vi "Parse Error XML.vi"(9 "Code Tag Value":string, 10 "Error XML":string, 11 "AWS Core":refnum<class "IoT Session.lvclass">) -> (1 "Error Description Override":string, 2 "Error Code":i32, 3 "Warning":bool)   [LabVIEW 2015, in "NI_AWS_IoT.lvlib" / "IoT Session.lvclass"]
uses:
  IoT Session.lvclass
  Core/HTTP Request/HTTP Request.lvclass
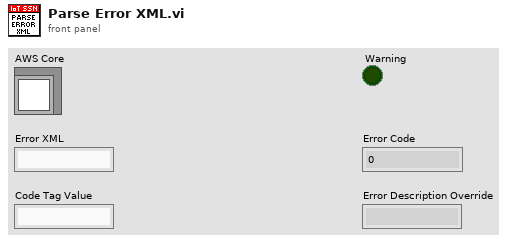
[diagram p1: front panel]
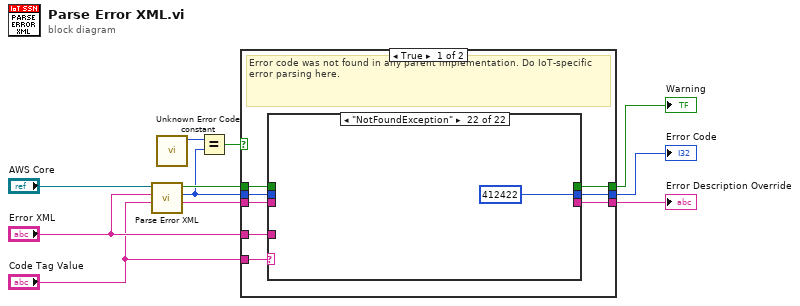
[diagram p0: block diagram]
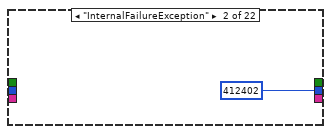
[diagram p3: hidden frame]
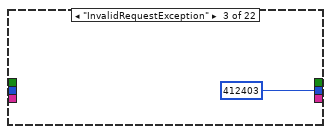
[diagram p4: hidden frame]
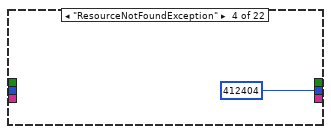
[diagram p5: hidden frame]
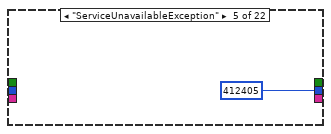
[diagram p6: hidden frame]
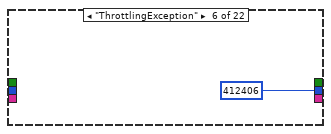
[diagram p7: hidden frame]
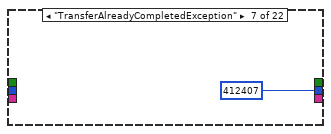
[diagram p8: hidden frame]
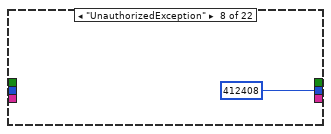
[diagram p9: hidden frame]
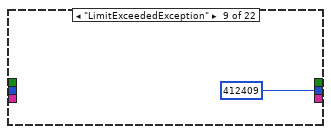
[diagram p10: hidden frame]
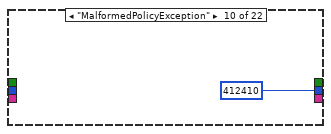
[diagram p11: hidden frame]
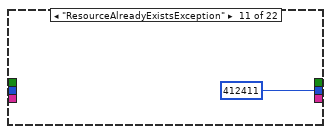
[diagram p12: hidden frame]
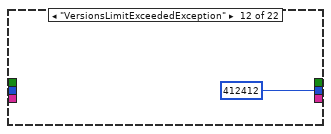
[diagram p13: hidden frame]
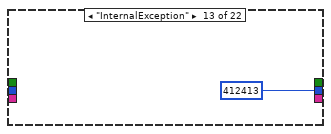
[diagram p14: hidden frame]
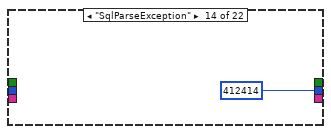
[diagram p15: hidden frame]
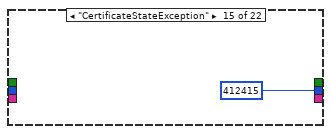
[diagram p16: hidden frame]
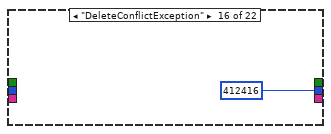
[diagram p17: hidden frame]
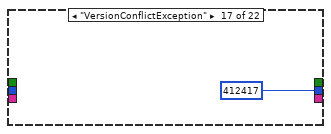
[diagram p18: hidden frame]
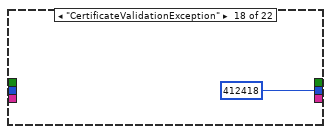
[diagram p19: hidden frame]
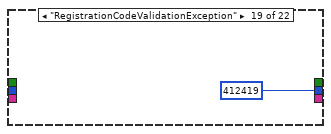
[diagram p20: hidden frame]
diagram:
  n1 = call-parent "Parse Error XML.vi"("Code Tag Value"="Code Tag Value", "Error XML"="Error XML", "AWS Core"="AWS Core") -> ("Error Description Override"=w6:string, "Error Code"=w7:i32, "Warning"=w8:bool)  [unwired: 6 in]
  n2 = call "Unknown Error Code constant.vi"() -> ("AWS Unknown Error Code value"=w10:i32)  [unwired: 11 in]
  n3 = Equal?(x=w10, y=w7) -> (x = y?=w9:bool)
  n4 = case shown="True" w9 {
    tunnel: w8 -> [w17 w46]
    tunnel: w6 -> [w15 w45]
    tunnel: [w14 w46] -> w1
    tunnel: [w12 w45] -> w3
    tunnel: [w13 w44] -> w2
    tunnel: "Error XML" -> [w18 _]
    tunnel: "Code Tag Value" -> [w19 _]
    tunnel: w7 -> [w16 w44]
    frame True {
      # "Error code was not found in any parent implementation. Do IoT-specific error parsing here."
      n5 = case shown="\"NotFoundException\"" w19 {
        tunnel: [w21 412402 412403 412404 412405 412406 412407 412408 412409 412410 412411 412412 412413 412414 412415 412416 412417 412418 412419 412420 412421 412422] -> w13
        tunnel: w18 -> [_ _ _ _ _ _ _ _ _ _ _ _ _ _ _ _ _ _ _ _ _ _]
        tunnel: w17 -> [w22 _ _ _ _ _ _ _ _ _ _ _ _ _ _ _ _ _ _ _ _ _]
        tunnel: w16 -> [w21 _ _ _ _ _ _ _ _ _ _ _ _ _ _ _ _ _ _ _ _ _]
        tunnel: w15 -> [w20 _ _ _ _ _ _ _ _ _ _ _ _ _ _ _ _ _ _ _ _ _]
        tunnel: [w22 _ _ _ _ _ _ _ _ _ _ _ _ _ _ _ _ _ _ _ _ _] -> w14
        tunnel: [w20 _ _ _ _ _ _ _ _ _ _ _ _ _ _ _ _ _ _ _ _ _] -> w12
        frame Default {
          # "Unknown error code, use default error from parent"
        }
        frame "InternalFailureException" {
        }
        frame "InvalidRequestException" {
        }
        frame "ResourceNotFoundException" {
        }
        frame "ServiceUnavailableException" {
        }
        frame "ThrottlingException" {
        }
        frame "TransferAlreadyCompletedException" {
        }
        frame "UnauthorizedException" {
        }
        frame "LimitExceededException" {
        }
        frame "MalformedPolicyException" {
        }
        frame "ResourceAlreadyExistsException" {
        }
        frame "VersionsLimitExceededException" {
        }
        frame "InternalException" {
        }
        frame "SqlParseException" {
        }
        frame "CertificateStateException" {
        }
        frame "DeleteConflictException" {
        }
        frame "VersionConflictException" {
        }
        frame "CertificateValidationException" {
        }
        frame "RegistrationCodeValidationException" {
        }
        frame "CertificateConflictException" {
        }
        frame "TransferConflictException" {
        }
        frame "NotFoundException" {
        }
      }
    }
    frame False {
      # "Parent method already assigned an error code"
    }
  }
  "Error Description Override" <- w3
  "Warning" <- w1
  "Error Code" <- w2
